vi "openHookViReference.vi"(8 "error in (no error)":errorcluster, 11 "TestSuite in":refnum<class "TestSuite.lvclass">) -> (0 "error out":errorcluster, 3 "TestSuite out":refnum<class "TestSuite.lvclass">)   [LabVIEW 2013, in "TestSuite.lvclass"]
uses:
  TestSuite.lvclass
  TestSuite.lvclass/TestSuite.ctl
  JKI Reuse/Filter Error Codes (Scalar)__jki_lib_error_handling -- VI Tester.vi
  Libraries/VITesterUtilities.lvlib
panel:
  # "JKI VI Tester for LabVIEW\nhttp://jkisoft.com/vi-tester\nCopyright (C) 2007-2009, JKI <info@jkisoft.com>\nALL RIGHTS RESERVED"
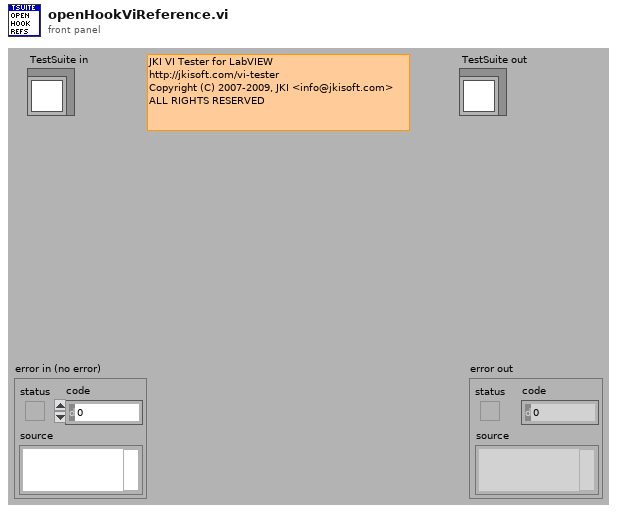
[diagram p1: front panel]
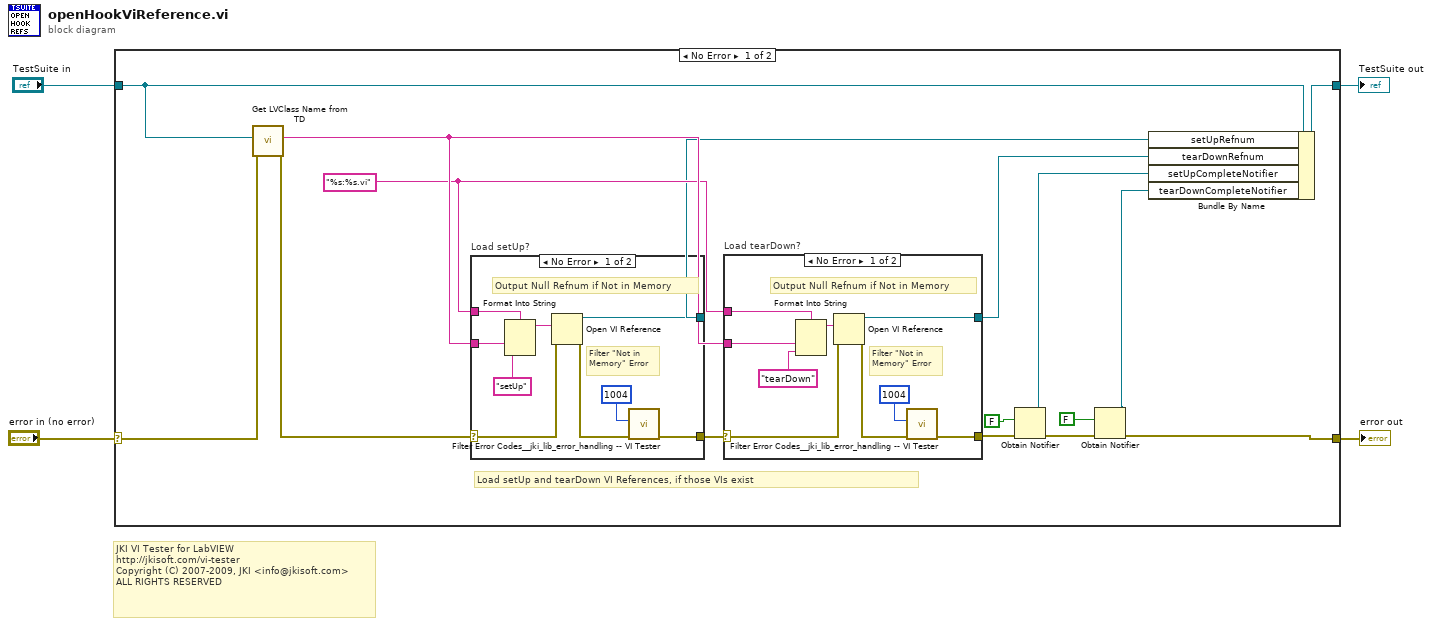
[diagram p0: block diagram]
diagram:
  # "JKI VI Tester for LabVIEW\nhttp://jkisoft.com/vi-tester\nCopyright (C) 2007-2009, JKI <info@jkisoft.com>\nALL RIGHTS RESERVED"
  n1 = case shown="No Error" "error in (no error)" {
    selector: "error in (no error)" -> [w18 w42]
    tunnel: [w7 w42] -> w3
    tunnel: [w20 w41] -> w1
    tunnel: "TestSuite in" -> [w19 w41]
    frame No Error {
      w16 = "%s:%s.vi" ("format string")
      # "Load setUp and tearDown VI References, if those VIs exist"
      n2 = call "Get LVClass Name from TD.vi"("error in"=w18, "Variant"=w19) -> ("error out"=w12:errorcluster, "LVClass Name"=w17:string)  [unwired: 8 in]
      n3 = case "Load setUp?" shown="No Error" w12 {
        selector: w12 -> [w34 w40]
        tunnel: [w37 _] -> w15
        tunnel: w16 -> [w36 _]
        tunnel: [w32 w40] -> w13
        tunnel: w17 -> [w35 _]
        frame No Error {
          # "Output Null Refnum if Not in Memory"
          # "Filter \"Not in Memory\" Error"
          n4 = Format Into String(format string=w36, w35, "setUp" ("input 2")) -> (resulting string=w38:string)  [unwired: 2 in, 1 out]
          n5 = Open VI Reference(vi path=w38, error in (no error)=w34) -> (vi reference=w37:refnum<vi>, error out=w33:errorcluster)  [unwired: 4 in]
          n6 = call-poly "Filter Error Codes__jki_lib_error_handling -- VI Tester.vi"("error in"=w33, "error code to filter"=1004) -> ("error out"=w32:errorcluster)  [unwired: 7 in, 2 out]
        }
        frame Error {
        }
      }
      n7 = case "Load tearDown?" shown="No Error" w13 {
        selector: w13 -> [w24 w30]
        tunnel: [w27 _] -> w14
        tunnel: w16 -> [w26 _]
        tunnel: [w22 w30] -> w9
        tunnel: w17 -> [w25 _]
        frame No Error {
          # "Output Null Refnum if Not in Memory"
          # "Filter \"Not in Memory\" Error"
          n8 = Format Into String(format string=w26, w25, "tearDown" ("input 2")) -> (resulting string=w28:string)  [unwired: 2 in, 1 out]
          n9 = Open VI Reference(vi path=w28, error in (no error)=w24) -> (vi reference=w27:refnum<vi>, error out=w23:errorcluster)  [unwired: 4 in]
          n10 = call-poly "Filter Error Codes__jki_lib_error_handling -- VI Tester.vi"("error in"=w23, "error code to filter"=1004) -> ("error out"=w22:errorcluster)  [unwired: 7 in, 2 out]
        }
        frame Error {
        }
      }
      n11 = Obtain Notifier(notification data type=FALSE, error in (no error)=w9) -> (notifier out=w6:refnum<notifier>, error out=w8:errorcluster)  [unwired: 2 in, 1 out]
      n12 = Obtain Notifier(notification data type=FALSE, error in (no error)=w8) -> (notifier out=w5:refnum<notifier>, error out=w7:errorcluster)  [unwired: 2 in, 1 out]
      n13 = Bundle By Name(cluster=w19, "setUpRefnum"=w15, "tearDownRefnum"=w14, "setUpCompleteNotifier"=w6, "tearDownCompleteNotifier"=w5) -> (w20:refnum<class "TestSuite.lvclass">)
    }
    frame Error {
    }
  }
  "error out" <- w3
  "TestSuite out" <- w1
